vi "Reg Key Constants.vi"() -> (0 "Default Templates Folder":path, 1 "String Value Name":string, 2 "Subkey Path":string, 3 "Root Key":T1=enum."HKEY_CURRENT_USER")   [LabVIEW 2022 SP3]
doc: "<add documentation here>"
uses:
  <vilib>/registry/registry.llb/Registry RtKey.ctl
  <vilib>/Utility/sysdir.llb/System Directory Type.ctl
panel:
  # "Development\nControls or indicators that are useful for development or testing, but which are not outputs of the VI."
  # "Input\nInputs to the VI"
  # "Output\nOutputs of the VI"
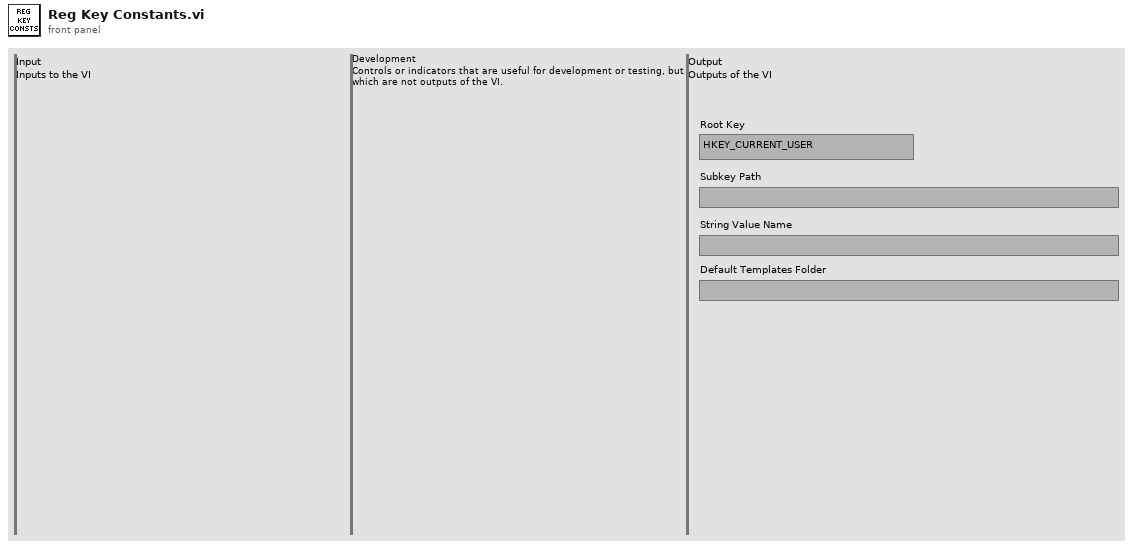
[diagram p1: front panel]
types:
  T1 = typedef "Registry RtKey.ctl" = enum32{"HKEY_CLASSES_ROOT", "HKEY_CURRENT_USER", "HKEY_LOCAL_MACHINE", "HKEY_USERS", "HKEY_PERFORMANCE_DATA", "HKEY_CURRENT_CONFIG", "HKEY_DYN_DATA"}
  T2 = typedef "System Directory Type.ctl" = i32
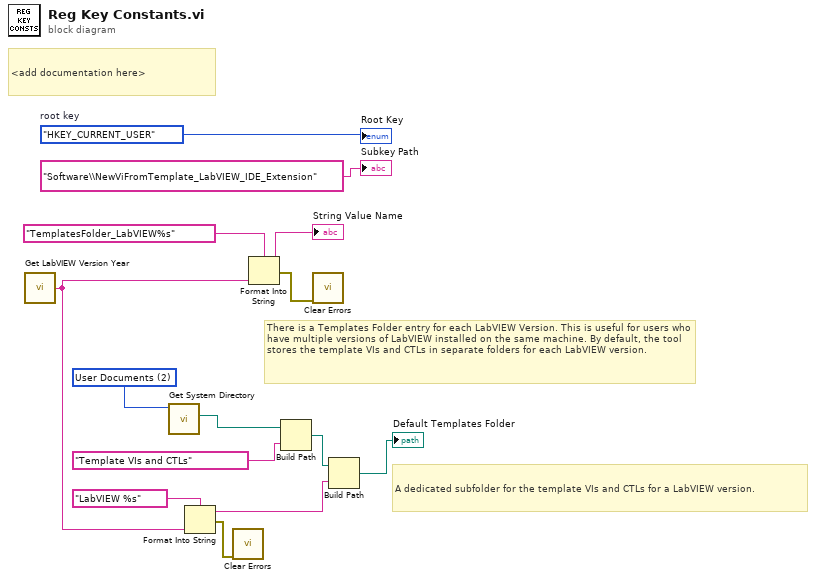
[diagram p0: block diagram]
diagram:
  w13 = T2 2 items=["User Home"=0, "User Desktop"=1, "User Documents"=2, "User Application Data"=3, "User Preferences"=4, "User Temporary"=5, "Public Documents"=6, "Public Application Data"=7, "Public Preferences"=8, "Public Cache"=13, "System Core Libraries"=9, "System Installed Libraries"=10, "Application Files"=11, "Boot Volume Root"=12] ("system directory type")
  w14 = Registry_RtKey."HKEY_CURRENT_USER"  # root key
  # "A dedicated subfolder for the template VIs and CTLs for a LabVIEW version."
  # "There is a Templates Folder entry for each LabVIEW Version. This is useful for users who have multiple versions of LabVIEW installed on the same machine. By default, the tool stores the template VIs and CTLs in separate folders for each LabVIEW version."
  # "<add documentation here>"
  n1 = call "Get LabVIEW Version Year.vi"() -> ("LabVIEW Version Year"=w4:string)
  n2 = call <vilib>:"Get System Directory.vi"("system directory type"=w13) -> ("system directory"=w12:path)  [unwired: 10 in]
  n3 = Format Into String(format string="LabVIEW %s", w4) -> (resulting string=w5:string, error out=w3:errorcluster)  [unwired: 2 in]
  n4 = call <vilib>:"Clear Errors.vi"("error in (no error)"=w3) -> ()  [unwired: 5 in, 2 out]
  n5 = Format Into String(format string="TemplatesFolder_LabVIEW%s", w4) -> (resulting string=→"String Value Name":string, error out=w10:errorcluster)  [unwired: 2 in]
  n6 = Build Path(base path=w12, name or relative path="Template VIs and CTLs") -> (appended path=w2:path)
  n7 = call <vilib>:"Clear Errors.vi"("error in (no error)"=w10) -> ()  [unwired: 5 in, 2 out]
  n8 = Build Path(base path=w2, name or relative path=w5) -> (appended path=→"Default Templates Folder":path)
  "Subkey Path" <- "Software\\NewViFromTemplate_LabVIEW_IDE_Extension"
  "Root Key" <- w14
